vi "CTRE_Phoenix_MotorController_GetParameter.vi"(8 "error in":errorcluster, 10 "Parameters":T1=1 items=["eOnBoot_BrakeMode"=31, "eQuadFilterEn"=91, "eStatusFramePeriod"=300, "eOpenLoopRamp"=301, "eClosedLoopRamp"=302, "eNeutralDeadband"=303, "ePeakPosOutput"=305, "eNominalPosOutput"=306, "ePeakNegOutput"=307, "eNominalNegOutput"=308, "eProfileParamSlot_P"=310, "eProfileParamSlot_I"=311, "eProfileParamSlot_D"=312, "eProfileParamSlot_F"=313, "eProfileParamSlot_IZone"=314, "eProfileParamSlot_AllowableErr"=315, "eProfileParamSlot_MaxIAccum"=316, "eClearPositionOnLimitF"=320, "eClearPositionOnLimitR"=321, "eClearPositionOnQuadIdx"=322, "eSampleVelocityPeriod"=325, "eSampleVelocityWindow"=326, "eFeedbackSensorType"=330, "eSelectedSensorPosition"=331, "eForwardSoftLimitThreshold"=340, "eReverseSoftLimitThreshold"=341, "eForwardSoftLimitEnable"=342, "eReverseSoftLimitEnable"=343, "eNominalBatteryVoltage"=350, "eBatterVoltageFilterSize"=351, "eContinuousCurrentLimitAmps"=360, "eContinuousCurrentLimitMs"=361, "ePeakCurrentLimitAmps"=362, "eClosedLoopIAccum"=370, "eCustomParam"=380, "eStickyFaults"=390, "eAnalogPosition"=400, "eQuadraturePosition"=401, "ePulseWidthPosition"=402, "eMotMag_Accel"=410, "eMotMag_VelCruise"=411, "eLimitSwitchSelect"=421, "eLimitSwitchNormClosed"=422, "eLimitSwitchDisabled"=423, "eLimitSwitchDisabledNeutralOnLOS"=424, "eLimitRemoteFilter_IDValue"=430, "eLimitRemoteFilter_IDMask"=431, "eLimitRemoteFilter_BitPos"=432, "eLimitRemoteFilter_TimeoutMs"=433], 11 "MotorControlDevRef":T2={"DeviceStatus"={"status"=FALSE, "code"=0, "source"=""}, "Type"=enum."PWM", "PWM"={"PWM Channel"=enum."Invalid", "DeadBand"={"Name"="", "maxPositivePwm"=0, "minPositivePwm"=0, "centerPwm"=0, "maxNegativePwm"=0, "minNegativePwm"=0, "angularRange"=0}}, "CAN"={"Device Number"=0, "SetOutput VI Ref"=variant(enum8{"Percent VBus", "Current", "Speed", "Position", "Voltage"} enum."Percent VBus"), "GetOutput VI Ref"=variant(refnum<k1> refnum), "Enable VI Ref"=variant(dbl 12.0), "Disable VI Ref"=variant(enum8{"Percent VBus", "Speed", "Position", "Slave", "Unchanged / Invalid", "Voltage Compensation", "Current", "Motion Profile"} enum."Percent VBus"), "Data"=variant}, "Invert"=FALSE}) -> (0 "error out":errorcluster, 2 "value":sgl, 3 "MotorControlDevRef":T2={"DeviceStatus"={"status"=FALSE, "code"=0, "source"=""}, "Type"=enum."PWM", "PWM"={"PWM Channel"=enum."Invalid", "DeadBand"={"Name"="", "maxPositivePwm"=0, "minPositivePwm"=0, "centerPwm"=0, "maxNegativePwm"=0, "minNegativePwm"=0, "angularRange"=0}}, "CAN"={"Device Number"=0, "SetOutput VI Ref"=variant(enum8{"Percent VBus", "Current", "Speed", "Position", "Voltage"} enum."Percent VBus"), "GetOutput VI Ref"=variant(refnum<k1> refnum), "Enable VI Ref"=variant(dbl 12.0), "Disable VI Ref"=variant(enum8{"Percent VBus", "Speed", "Position", "Slave", "Unchanged / Invalid", "Voltage Compensation", "Current", "Motion Profile"} enum."Percent VBus"), "Data"=variant}, "Invert"=FALSE})   [LabVIEW 2016]
doc: "Returns the selected parameter value."
uses:
  <vilib>/Rock Robotics/WPI/MotorControl/WPI_MotorControlDeviceRef.ctl
  <vilib>/Rock Robotics/WPI/MotorControl/WPI_MotorControlType.ctl
  <vilib>/Rock Robotics/SystemInterfaces/DIO/FPGA_DIOPWMChannel.ctl
  <vilib>/Rock Robotics/WPI/PWM/WPI_PWMDeadband.ctl
  Controls/CTRE_Phoenix_Params.ctl
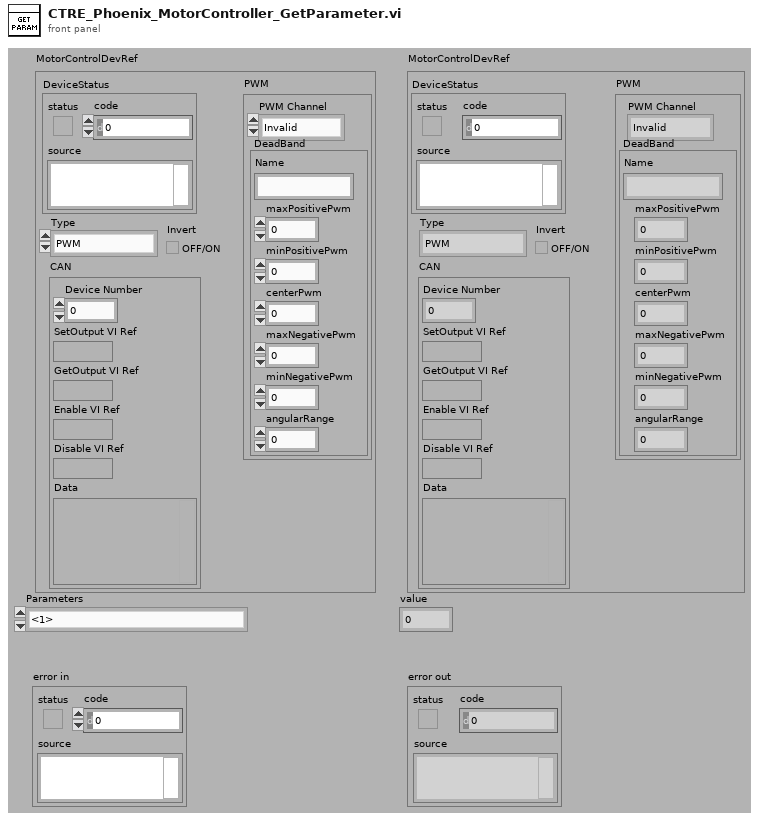
[diagram p1: front panel]
types:
  T1 = typedef "CTRE_Phoenix_Params.ctl" = u16
  T2 = typedef "WPI_MotorControlDeviceRef.ctl" = cluster{"DeviceStatus":errorcluster, "Type":T3, "PWM":cluster{"PWM Channel":T4, "DeadBand":T5}, "CAN":cluster{"Device Number":u8, "SetOutput VI Ref":variant, "GetOutput VI Ref":variant, "Enable VI Ref":variant, "Disable VI Ref":variant, "Data":variant}, "Invert":bool}
  T3 = typedef "WPI_MotorControlType.ctl" = enum16{"PWM", "CAN"}
  T4 = typedef "FPGA_DIOPWMChannel.ctl" = enum8{"PWM 0", "PWM 1", "PWM 2", "PWM 3", "PWM 4", "PWM 5", "PWM 6", "PWM 7", "PWM 8", "PWM 9", "PWM MXP 0", "PWM MXP 1", "PWM MXP 2", "PWM MXP 3", "PWM MXP 4", "PWM MXP 5", "PWM MXP 6", "PWM MXP 7", "PWM MXP 8", "PWM MXP 9", "Invalid"}
  T5 = typedef "WPI_PWMDeadband.ctl" = cluster{"Name":string, "maxPositivePwm":i32, "minPositivePwm":i32, "centerPwm":i32, "maxNegativePwm":i32, "minNegativePwm":i32, "angularRange":u16}
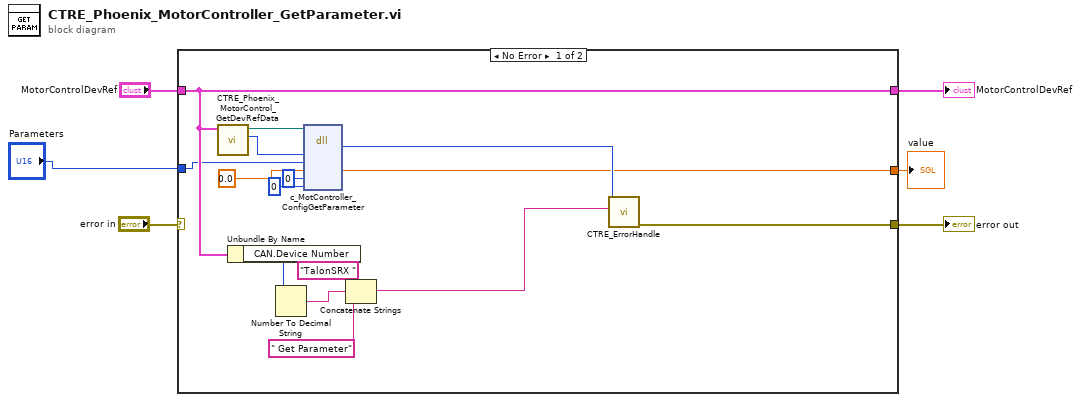
[diagram p0: block diagram]
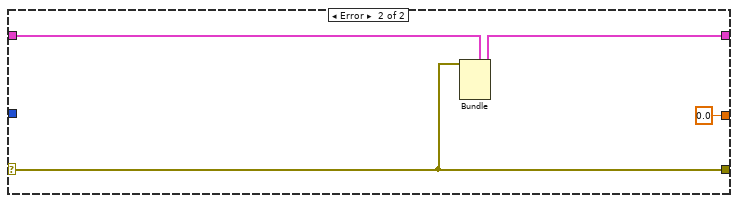
[diagram p2: hidden frame]
diagram:
  n1 = case shown="No Error" "error in" {
    selector: "error in" -> [_ w24]
    tunnel: "MotorControlDevRef" -> [w14 w25]
    tunnel: [w21 w24] -> w5
    tunnel: [w14 w23] -> w3
    tunnel: "Parameters" -> [w11 _]
    tunnel: [w7 sgl 0.0 ("value")] -> w1
    frame No Error {
      n2 = call "CTRE_Phoenix_MotorControl_GetDevRefData.vi"("MotorControlDevRef"=w14) -> ("handle"=w12:u64, "Library"=w13:path)  [unwired: 4 in, 5 out]
      n3 = Unbundle By Name(w14) -> ("CAN.Device Number"=w17:u8)
      n4 = Number To Decimal String(number=w17) -> (decimal integer string=w19:string)  [unwired: 1 in]
      n5 = dll-call lib="?" fn="c_MotController_ConfigGetParameter"(path in=w13, "handle"=w12, "param"=w11, "value"=sgl 0.0, "ordinal"=0, "timeoutMs"=0) -> ("return type"=w16:i32, "value"=w7:sgl)  [unwired: 6 in, 2 out]
      n6 = Concatenate Strings("TalonSRX " ("string"), w19, " Get Parameter" ("string")) -> (w15:string)
      n7 = call "CTRE_ErrorHandle.vi"("origin"=w15, "code"=w16) -> ("error out"=w21:errorcluster)  [unwired: 9 in]
    }
    frame Error {
      n8 = Bundle(cluster=w25, "DeviceStatus"=w24) -> (w23:T2)  [unwired: 4 in]
    }
  }
  "MotorControlDevRef" <- w3
  "error out" <- w5
  "value" <- w1
